vi "setError.vi"(1 "error":errorcluster) -> ()   [LabVIEW 2010]
uses:
  ErrorsGlobal.vi
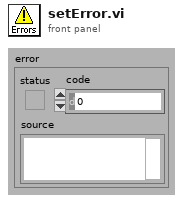
[diagram p1: front panel]
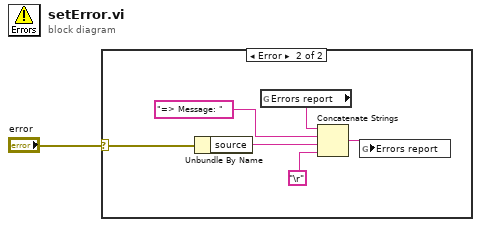
[diagram p0: block diagram]
diagram:
  n1 = case shown="Error" "error" {
    selector: "error" -> [_ w7]
    frame No Error {
    }
    frame Error {
      n2 = Unbundle By Name(w7) -> ("source"=w5:string)
      n3 = global read "ErrorsGlobal.vi" "Errors report"() -> (w3:string)
      n4 = Concatenate Strings(w3, "=> Message: " ("string"), w5, "\r") -> (w4:string)
      n5 = global write "ErrorsGlobal.vi" "Errors report"(w4) -> ()
    }
  }
